vi "ble_string2hex.vi"(11 "HEX string IN":string) -> (3 "Byte Array IN (index0 LS byte)":u8[](array[numeric]) format="%02x")   [LabVIEW 2017]
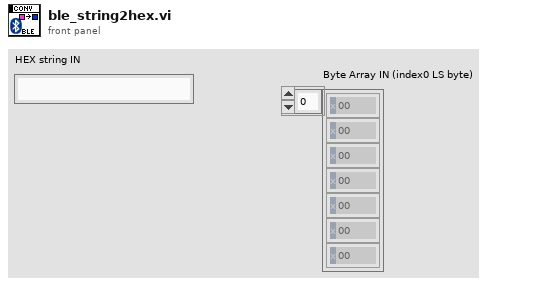
[diagram p1: front panel]
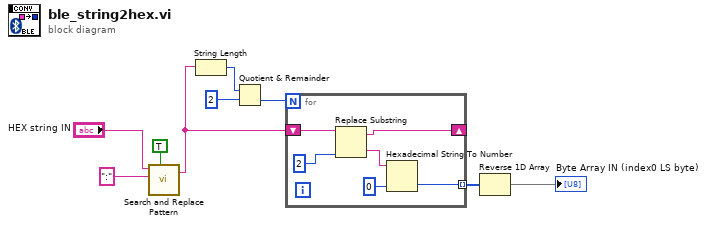
[diagram p0: block diagram]
diagram:
  n1 = call <vilib>:"Search and Replace Pattern.vi"("string"="HEX string IN", "regular expression (\"\")"=":" ("regular expression (\"\")"), "replace all? (F)"=TRUE) -> ("result string"=w4:string)  [unwired: 2 in, 1 out]
  n2 = String Length(string=w4) -> (length=w3:i32)
  n3 = Quotient & Remainder(x=w3, y=2 ("offset (0)")) -> (floor(x/y)=w1:i32)  [unwired: 1 out]
  n4 = for {
    N: w1 -> [_]
    shift-right: [w10] -> _
    shift-left: w4 -> [w15]
    tunnel: [w12] -> w9 mode=indexing
    n5 = Replace Substring(2:2 ("offset (0)"), 5:w15) -> (0:w11:string, 1:w10:string)  [unwired: 2 in]
    n6 = Hexadecimal String To Number(string=w11, default (0uL)=u8 0 ("default (0 U32)")) -> (number=w12:u8)  [unwired: 1 in, 1 out]
  }
  n7 = Reverse 1D Array(array=w9) -> (reversed array=→"Byte Array IN (index0 LS byte)":u8[])
